vi "receiver_daq.vi"() -> (0 "Boolean":bool)   [LabVIEW 2013]
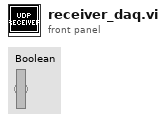
[diagram p1: front panel]
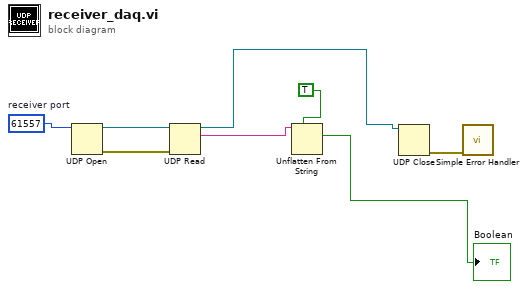
[diagram p0: block diagram]
diagram:
  w3 = u16 61557  # receiver port
  n1 = UDP Open(11:w3) -> (port=w4:refnum<k16>, 0:w5:errorcluster)  [unwired: 4 in, 1 out]
  n2 = UDP Read(connection ID=w4, 8:w5) -> (data out=w6:string, 3:w8:refnum<k16>)  [unwired: 1 in, 4 out]
  n3 = Unflatten From String(type=TRUE, binary string=w6) -> (value=→"Boolean":bool)  [unwired: 3 in, 2 out]
  n4 = UDP Close(connection ID=w8) -> (error out=w7:errorcluster)  [unwired: 1 in, 1 out]
  n5 = call <vilib>:"Simple Error Handler.vi"("error in (no error)"=w7) -> ()  [unwired: 1 in, 8 out]
